vi "Write Status 1D.vi"(8 "error in (no error)":errorcluster, 10 "statuses":T1[](array[typedef]) {"period" format="%d us"; "duration" format="%d us"}, 11 "status pointer in":refnum<class "Status Pointer.lvclass">) -> (0 "error out":errorcluster, 3 "status pointer out":refnum<class "Status Pointer.lvclass">)   [LabVIEW 2021, in "DSF Core.lvlib" / "Status Pointer.lvclass"]
uses:
  Status Pointer.lvclass
  C:/Program Files/National Instruments/LabVIEW 2021/vi.lib/NI/Memory Manager/Classes/Pointer/Pointer.lvclass
  Status Data.ctl
  <vilib>/NI/Memory Manager/Classes/Pointer/Pointer.lvclass/Pointer.ctl
  <vilib>/NI/Memory Manager/Classes/Pointer/Errors.vi
  <vilib>/NI/Memory Manager/Classes/Pointer/Out of Bounds.vi
  <vilib>/NI/Memory Manager/Classes/Pointer/Get Size.vi
  <vilib>/NI/Memory Manager/Classes/Pointer/Null Pointer.vi
  <vilib>/NI/Memory Manager/Classes/Pointer/Is Null.vi
  <vilib>/NI/Memory Manager/VIs/Write String to Source.vi
  <vilib>/NI/Memory Manager/Classes/Pointer/Write Pointer Size to Error.vi
  <vilib>/NI/Memory Manager/Classes/Pointer/Create Error.vi
  <vilib>/NI/Memory Manager/VIs/Write Numeric to Source.vi
  <vilib>/NI/Memory Manager/VIs/Write Numeric Scalar to Source (Base10 U64).vi
  <vilib>/NI/Memory Manager/VIs/New Error Cluster.vi
  <vilib>/NI/Memory Manager/VIs/New Error Cluster (512B).vi
  <vilib>/NI/Memory Manager/VIs/Set Error Status.vi
  <vilib>/NI/Memory Manager/VIs/Set Error Code.vi
  <vilib>/NI/Memory Manager/VIs/Set Error Source.vi
  <vilib>/NI/Memory Manager/Constants/Constants.vi
  <vilib>/NI/Memory Manager/Constants/Library Name.vi
  <vilib>/NI/Memory Manager/Classes/Pointer/Pointer Error Info.vi
  <vilib>/NI/Memory Manager/Constants/Pointer Class Name.vi
  <vilib>/NI/Memory Manager/Classes/Pointer/Pointer.lvclass
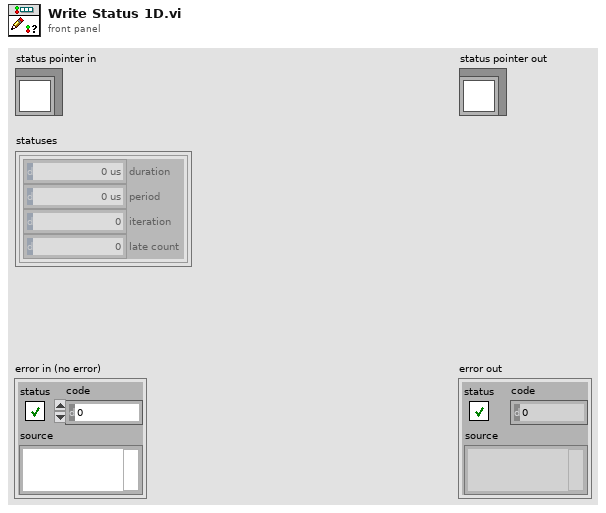
[diagram p1: front panel]
types:
  T1 = typedef "DSF Core.lvlib/Status Pointer.lvclass/Status Data.ctl" = cluster{"duration":u64, "period":u64, "iteration":u64, "late count":u64}
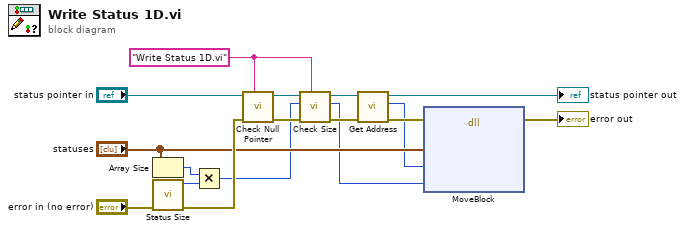
[diagram p0: block diagram]
diagram:
  w11 = "Write Status 1D.vi" ("source vi name")
  n1 = Array Size(array="statuses") -> (size(s)=w6:i32)
  n2 = call "Status Size.vi"("error in (no error)"="error in (no error)") -> ("error out"=w8:errorcluster, "size"=w7:u64)  [unwired: 9 in]
  n3 = Multiply(x=w6, y=w7) -> (x*y=w3:u64)
  n4 = call <vilib>:"Check Null Pointer.vi"("source vi name"=w11, "error in (no error)"=w8, "Pointer in"="status pointer in") -> ("error out"=w9:errorcluster, "Pointer out"=w14:refnum<class "Status Pointer.lvclass">)  [unwired: 7 in]
  n5 = call <vilib>:"Check Size.vi"("source vi name"=w11, "error in (no error)"=w9, "required size"=w3, "Pointer in"=w14) -> ("error out"=w5:errorcluster, "required size out"=w2:u64, "Pointer out"=w12:refnum<class "Status Pointer.lvclass">)  [unwired: 5 in]
  n6 = call <vilib>:"Get Address.vi"("Pointer in"=w12) -> ("address"=w1:u64, "Pointer out"=→"status pointer out":refnum<class "Status Pointer.lvclass">)  [unwired: 9 in]
  n7 = dll-call lib="LabVIEW" fn="MoveBlock"(error in=w5, "src"="statuses", "dst"=w1, "size"=w2) -> (error out=→"error out":errorcluster)  [unwired: 6 in, 1 out]
